vi "Scopeset_diag.vi"(0 "Ref_MLD measurement":dbl[][](array[numeric]), 1 "V/div in B":dbl(knob) scale=10.0..0.01, 3 "Second":bool, 4 "AC?":bool, 5 "V/div in A":dbl(knob) scale=10.0..0.01, 7 "level B":dbl(slide) scale=-1.0..1.0, 8 "level A":dbl(slide) scale=-1.0..1.0, 9 "dt":dbl) -> (12 "UP":bool, 13 "Down":bool, 14 "V/div out":dbl, 15 "Waveform":waveform(dbl), 16 "Ref_MLD_triggered":dbl[][](array[numeric]), 17 "levelB":dbl, 18 "MLD_mean":dbl format="%0.2f", 20 "Scale Max":dbl, 21 "Scale Min":dbl, 23 "levelA":dbl, 24 "First Rising edge index":i32, 25 "Array":waveform(dbl)[](array[waveform]), 27 "Frequency":dbl)   [LabVIEW 2015]
uses:
  <vilib>/Analysis/baseanly.llb/Mean (DBL).vi
  <vilib>/Analysis/NI_AALBase.lvlib
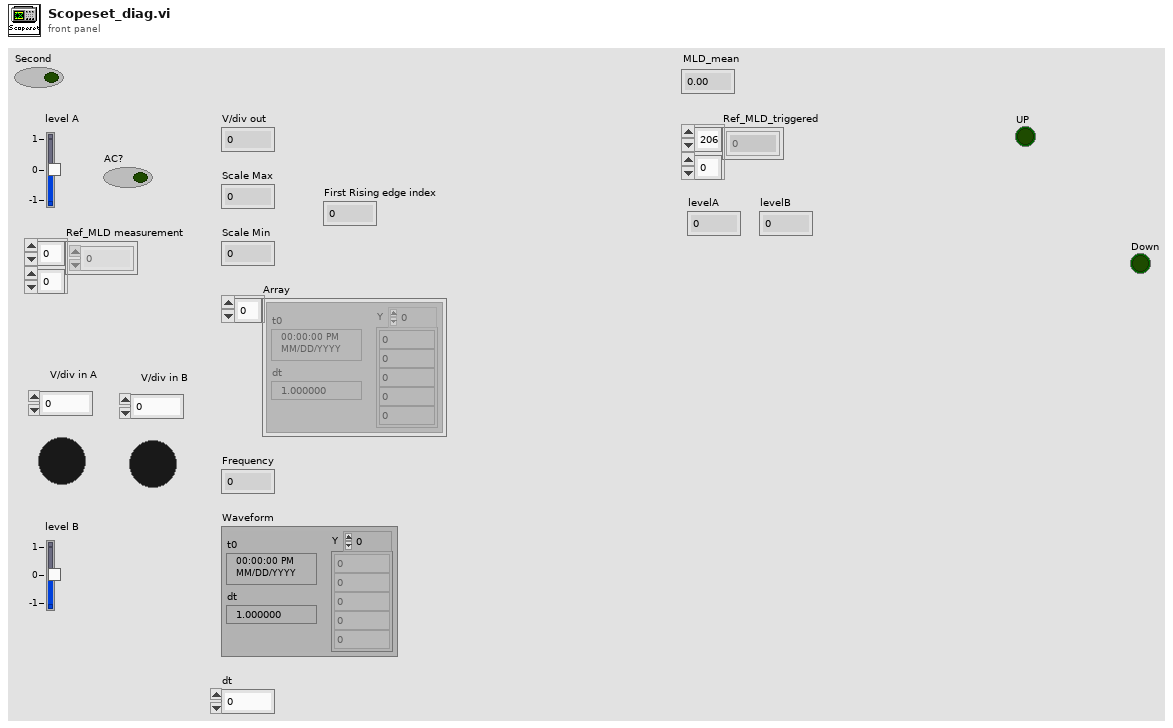
[diagram p1: front panel]
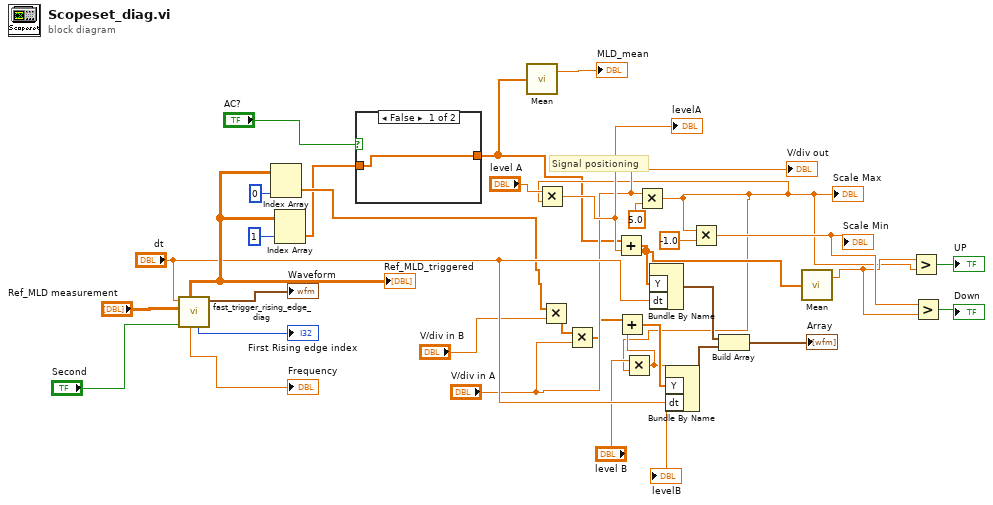
[diagram p0: block diagram]
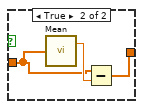
[diagram p2: hidden frame]
diagram:
  # "Signal positioning"
  n1 = call "fast_trigger_rising_edge_diag.vi"("Second"="Second", "Ref_MLD measurement"="Ref_MLD measurement", "dt in"="dt") -> ("Waveform"=→"Waveform":waveform(dbl), "First Rising edge index"=→"First Rising edge index":i32, "Frequency"=→"Frequency":dbl, "Ref_MLD_triggered"=w23:dbl[][])  [unwired: 5 in]
  "Ref_MLD_triggered" <- w23
  n2 = Index Array(array=w23, index (col)=0 ("disabled index (col)")) -> (element=w20:dbl[])  [unwired: 1 in]
  n3 = Index Array(array=w23, index (col)=1 ("disabled index (col)")) -> (element=w11:dbl[])  [unwired: 1 in]
  n4 = case shown="False" "AC?" {
    tunnel: w11 -> [w35 w37]
    tunnel: [w35 w36] -> w2
    frame False {
    }
    frame True {
      n5 = call-poly <vilib>:"Mean.vi"("X"=w37) -> ("mean"=w38:dbl)  [unwired: 1 out]
      n6 = Subtract(x=w37, y=w38) -> (x-y=w36:dbl[])
    }
  }
  n7 = call-poly <vilib>:"Mean.vi"("X"=w2) -> ("mean"=→"MLD_mean":dbl)  [unwired: 1 out]
  n8 = Multiply(x=w20, y="V/div in B") -> (x*y=w14:dbl[])
  n9 = Multiply(x=w14, y="V/div in A") -> (x*y=w12:dbl[])
  n10 = Multiply(x="V/div in A", y=5.0) -> (x*y=w4:dbl)
  "Scale Max" <- w4
  n11 = Multiply(x="level A", y=w4) -> (x*y=w16:dbl)
  "levelA" <- w16
  n12 = Add(x=w2, y=w16) -> (x+y=w9:dbl[])
  n13 = Multiply(x="level B", y=w4) -> (x*y=w18:dbl)
  "levelB" <- w18
  n14 = Add(x=w12, y=w18) -> (x+y=w21:dbl[])
  n15 = Bundle By Name("Y"=w9, "dt"="dt") -> (w31:waveform(dbl))  [unwired: 1 in]
  n16 = Bundle By Name("Y"=w21, "dt"="dt") -> (w29:waveform(dbl))  [unwired: 1 in]
  n17 = Multiply(x=w4, y=-1.0) -> (x*y=w7:dbl)
  "Scale Min" <- w7
  n18 = Build Array(w31, w29) -> (→"Array":waveform(dbl)[])
  n19 = call-poly <vilib>:"Mean.vi"("X"=w9) -> ("mean"=w5:dbl)  [unwired: 1 out]
  n20 = Greater?(x=w5, y=w4) -> (0:→"UP":bool)
  n21 = Greater?(x=w7, y=w5) -> (0:→"Down":bool)
  "V/div out" <- "V/div in A"
